vi "DB Request Calibration Points.vi"(8 "error in (no error)":errorcluster, 9 "UI Device Type":T1, 10 "UI List Type":T2, 11 "Database in":refnum<queue>) -> (0 "error out":errorcluster, 2 "Results":string[][](array[string]), 3 "Database out":refnum<queue>)   [LabVIEW 2026, in "Analysis.lvlib"]
uses:
  Analysis/Analysis.lvlib
  support/Architecture/Message Queue/Message Queue.lvlib
  support/Architecture/Message Queue/Enqueue Message (Single).vi
  controls/UI/UI List Type.ctl
  controls/UI/Data Entity.ctl
  Settings/Settings.lvlib
  controls/Messaging Payloads/DB Query Request 2D Payload.ctl
  Database.lvlib
  support/Architecture/Message Queue/Message Cluster.ctl
panel:
  in  "Test Run ID":i32
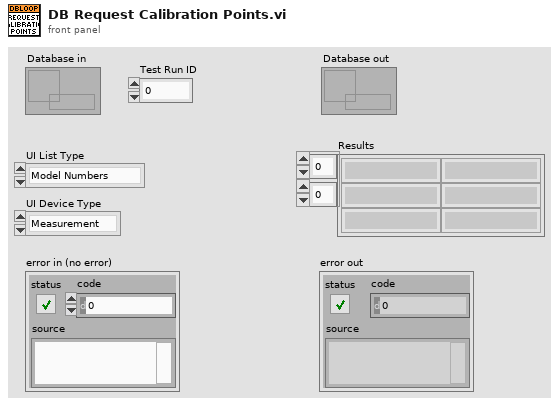
[diagram p1: front panel]
types:
  T1 = typedef "Settings.lvlib/Data Entity.ctl" = enum16{"Measurement", "Controller"}
  T2 = typedef "UI List Type.ctl" = enum16{"Model Numbers", "Serial Numbers", "Operators", "Calibration Points", "Start Run Times"}
  T3 = typedef "Database.lvlib/DB Query Request 2D Payload.ctl" = cluster{"Notifier":refnum<notifier>, "UI List Type":T2, "UI Device Type":T1, "Identifier":i32}
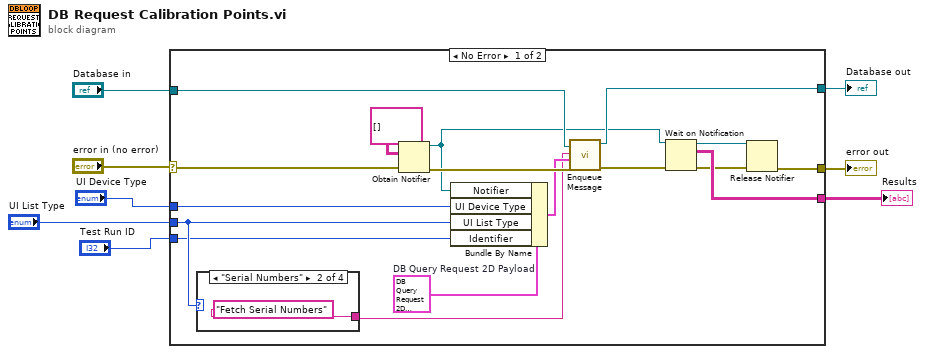
[diagram p0: block diagram]
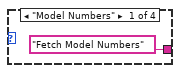
[diagram p2: hidden frame]
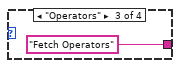
[diagram p3: hidden frame]
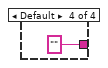
[diagram p4: hidden frame]
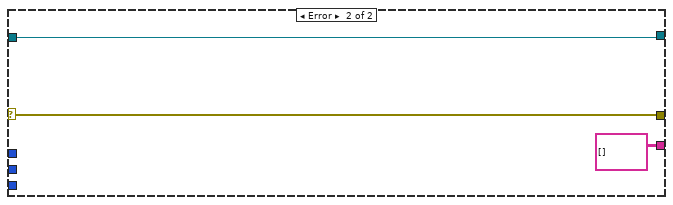
[diagram p5: hidden frame]
diagram:
  n1 = case shown="No Error" "error in (no error)" {
    selector: "error in (no error)" -> [w16 w31]
    tunnel: [w25 string[][] []] -> w2
    tunnel: [w24 w32] -> w8
    tunnel: "Database in" -> [w23 w32]
    tunnel: [w22 w31] -> w6
    tunnel: "UI List Type" -> [w11 _]
    tunnel: "UI Device Type" -> [w10 _]
    tunnel: "Test Run ID" -> [w9 _]
    frame No Error {
      w15 = T3 {"Notifier"=refnum, "UI List Type"=enum."Model Numbers", "UI Device Type"=enum."Measurement", "Identifier"=0}  # DB Query Request 2D Payload
      n2 = case shown="\"Serial Numbers\"" w11 {
        tunnel: ["Fetch Model Numbers" "Fetch Serial Numbers" "Fetch Operators" ""] -> w13
        frame "Model Numbers" {
        }
        frame "Serial Numbers" {
        }
        frame "Operators" {
        }
        frame Default {
        }
      }
      n3 = Obtain Notifier(notification data type=string[][] [], error in (no error)=w16) -> (notifier out=w12:refnum<notifier>, error out=w18:errorcluster)  [unwired: 2 in, 1 out]
      n4 = Bundle By Name(cluster=w15, "Notifier"=w12, "UI Device Type"=w10, "UI List Type"=w11, "Identifier"=w9) -> (w14:T3)
      n5 = call-poly "Enqueue Message.vi"("error in (no error)"=w18, "Message Data"=w14, "Message"=w13, "Message Queue"=w23) -> ("error out"=w19:errorcluster, "dup Message Queue"=w24:refnum<queue>)  [unwired: 6 in]
      n6 = Wait on Notification(notifier=w12, error in (no error)=w19) -> (notifier out=w21:refnum<notifier>, notification=w25:string[][], error out=w20:errorcluster)  [unwired: 2 in, 1 out]
      n7 = Release Notifier(notifier=w21, error in (no error)=w20) -> (error out=w22:errorcluster)  [unwired: 1 in, 2 out]
    }
    frame Error {
    }
  }
  "Results" <- w2
  "Database out" <- w8
  "error out" <- w6
